vi "cm2nm_save_sample.vi"() -> ()   [LabVIEW 2010]
uses:
  cm2nm_sample_set.ctl
  cm2nm_coordinate_information_v2.ctl
  <vilib>/Utility/xml.llb/Write to XML File(string).vi
panel:
  in  "Sample Set":T1={"CollectionOfPoints"=[{"MetaDataFile"=path "", "X"=50.1935, "Y"=19.379, "Group"=1, "Z"=0.0, "Rotation"=0.0, "Fiducial"=FALSE, "Magnification"=0.0, "Working_Distance"=0.0, "Notes"="", "Location Name/ID"="Interface_corrected", "OtherRelatedDataFiles"=[], "Available"=FALSE}, {"MetaDataFile"=path "", "X"=38.1101655, "Y"=26.3691263, "Group"=1, "Z"=0.0, "Rotation"=0.0, "Fiducial"=TRUE, "Magnification"=0.0, "Working_Distance"=0.0, "Notes"="", "Location Name/ID"="F1", "OtherRelatedDataFiles"=[], "Available"=TRUE}, {"MetaDataFile"=path "", "X"=43.2008536, "Y"=7.322264, "Group"=1, "Z"=0.0, "Rotation"=0.0, "Fiducial"=TRUE, "Magnification"=0.0, "Working_Distance"=0.0, "Notes"="", "Location Name/ID"="F3B", "OtherRelatedDataFiles"=[], "Available"=TRUE}, {"MetaDataFile"=path "", "X"=62.077256, "Y"=12.0875, "Group"=1, "Z"=0.0, "Rotation"=0.0, "Fiducial"=TRUE, "Magnification"=0.0, "Working_Distance"=0.0, "Notes"="", "Location Name/ID"="F5C", "OtherRelatedDataFiles"=[], "Available"=FALSE}, {"MetaDataFile"=path "", "X"=51.9658407, "Y"=19.1617677, "Group"=1, "Z"=0.0, "Rotation"=0.0, "Fiducial"=FALSE, "Magnification"=0.0, "Working_Distance"=0.0, "Notes"="", "Location Name/ID"="Corner_correcte_S1", "OtherRelatedDataFiles"=[], "Available"=FALSE}, {"MetaDataFile"=path "", "X"=51.947965, "Y"=19.1779565, "Group"=1, "Z"=0.0, "Rotation"=0.0, "Fiducial"=FALSE, "Magnification"=0.0, "Working_Distance"=0.0, "Notes"="", "Location Name/ID"="Corner_corrected_S2", "OtherRelatedDataFiles"=[], "Available"=FALSE}], "Instrument"=2, "CollectionFile"=path "/INL Macintosh/Users/timothymcjunkin/Desktop/Diffusion couple/JEOL 7000F SEM 9-3-10/Corrected_9-3-10.xlm", "Session Name/ID"="Correct_Abs_position", "SessionNotes"="EMSA images were taken off center so I May need to add the two together"} {"Instrument" items=["Unknown", "Phillips SEM IRC", "JEOL 7000F EML_MFC", "MXRD MFC"]; "CollectionOfPoints"."Rotation" min=-37480660.29033894 max=37480660.27288565}
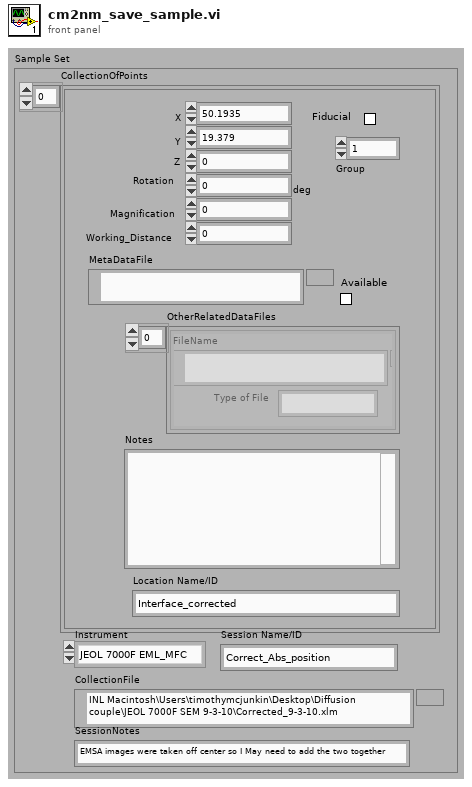
[diagram p1: front panel]
types:
  T1 = typedef "cm2nm_sample_set.ctl" = cluster{"CollectionOfPoints":T2[], "Instrument":u16, "CollectionFile":path, "Session Name/ID":string, "SessionNotes":string}
  T2 = typedef "cm2nm_coordinate_information_v2.ctl" = cluster{"MetaDataFile":path, "X":dbl, "Y":dbl, "Group":i32, "Z":dbl, "Rotation":dbl[unit], "Fiducial":bool, "Magnification":dbl, "Working_Distance":dbl, "Notes":string, "Location Name/ID":string, "OtherRelatedDataFiles":cluster{"Type of File":string, "FileName":path}[], "Available":bool}
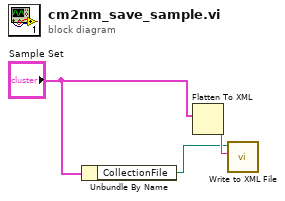
[diagram p0: block diagram]
diagram:
  n1 = Unbundle By Name("Sample Set") -> ("CollectionFile"=w1:path)
  n2 = Flatten To XML(anything="Sample Set") -> (xml string=w3:string)
  n3 = call-poly <vilib>:"Write to XML File.vi"("XML Input"=w3, "XML File Path"=w1) -> ()  [unwired: 3 in, 7 out]
